vi "torque -- filename controller.vi"(7 "filename action":T2, 8 "Angle (deg) IN":dbl, 9 "Temperature (K) IN":dbl, 11 "String":string="30K_-45D_001_061513.dat") -> (0 "Angle (deg)":dbl=-45.0, 1 "Temperature (K)":dbl=30.0, 2 "file name regexp":string="(?:\\d+[Ss])?_?(\\d+)K_?([0-9\\+\\-\\.]+)(?:D|deg)?_.*?\\.dat", 3 "Ok?":bool, 4 "hash key":T1)   [LabVIEW 2012]
uses:
  torque -- filename action.ctl
  torque -- hash key.ctl
  <vilib>/regexp/Match Regular Expression.xnode
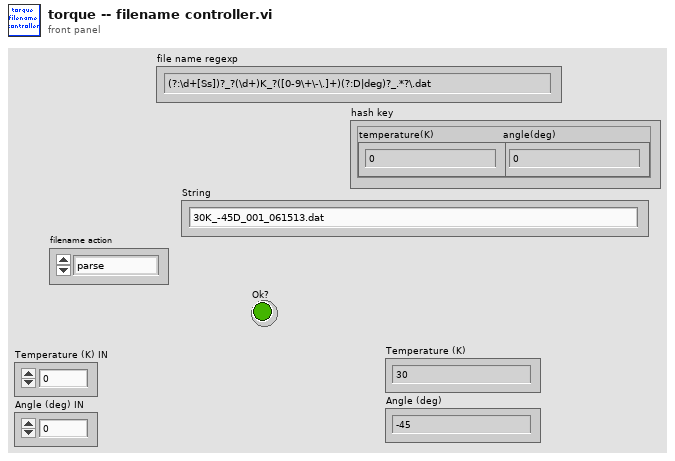
[diagram p1: front panel]
types:
  T1 = typedef "torque -- hash key.ctl" = cluster{"temperature(K)":dbl, "angle(deg)":dbl}
  T2 = typedef "torque -- filename action.ctl" = enum16{"parse", "build", "check"}
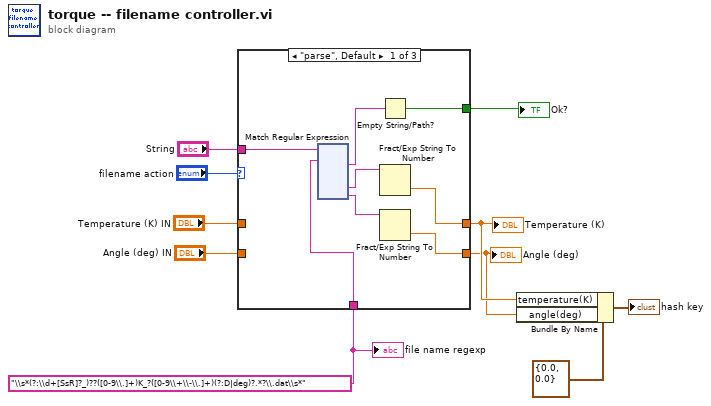
[diagram p0: block diagram]
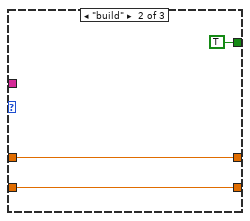
[diagram p2: hidden frame]
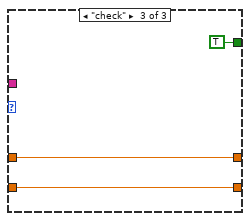
[diagram p3: hidden frame]
diagram:
  w8 = "\\s*(?:\\d+[SsR]?_)??([0-9\\.]+)K_?([0-9\\+\\-\\.]+)(?:D|deg)?.*?\\.dat\\s*" ("regular expression")
  n1 = case shown="\"parse\", Default" "filename action" {
    tunnel: "String" -> [w18 _ _]
    tunnel: w8 -> [w17 _ _]
    tunnel: [w15 w135 w138] -> w3
    tunnel: [w13 w134 w137] -> w2
    tunnel: "Temperature (K) IN" -> [_ w135 w138]
    tunnel: "Angle (deg) IN" -> [_ w134 w137]
    tunnel: [w11 TRUE TRUE] -> w5
    frame "parse", Default {
      n2 = xnode "Match Regular Expression"("input string"=w18, "regular expression"=w17) -> ("after match"=w12:string, "submatch 1"=w16:string, "submatch 2"=w14:string)  [unwired: 4 in, 4 out]
      n3 = Empty String/Path?(string/path=w12) -> (empty?=w11:bool)
      n4 = Fract/Exp String To Number(string=w16) -> (number=w15:dbl)  [unwired: 3 in, 1 out]
      n5 = Fract/Exp String To Number(string=w14) -> (number=w13:dbl)  [unwired: 3 in, 1 out]
    }
    frame "build" {
    }
    frame "check" {
    }
  }
  "Temperature (K)" <- w3
  "Angle (deg)" <- w2
  "Ok?" <- w5
  n6 = Bundle By Name(cluster=T1 {"temperature(K)"=0.0, "angle(deg)"=0.0} ("hash key"), "temperature(K)"=w3, "angle(deg)"=w2) -> (→"hash key":T1)
  "file name regexp" <- w8
